vi "INLScan.vi"() -> ()   [LabVIEW 2014]
uses:
  Agilent34401A/FGV.ctl
  Agilent34401A/Agilent34401AData.ctl
  Host API/Controls/FPGA Reference.ctl
  <vilib>/rvi/interface/nirviOpenFPGA/nirviOpenFPGA.xnode
  <vilib>/rvi/interface/nirviMethod/nirviMethod.xnode
  Host API/Controls/SPI Configuration Cluster.ctl
  <vilib>/rvi/interface/nirviCloseFPGA/nirviCloseFPGA.xnode
  FPGA Bitfiles/SPIExample_FPGATarget3_FPGASPIFPGATopLe_SKx8rjJlgp0.lvbitx
  FPGA/FPGA SPI_FPGA Top Level.vi
  <vilib>/rvi/errors/niLvFpgaMergeErrorWithErrorCode.vi
panel:
  out "act rep.":i32
  in  "repetitions":i32
  out "KepcoStep [V]":ext
  out "DAC step [V]":ext format="%#_10g"
  out "StepSize":u32 max=262143 format="%0d"
  out "INL":dbl
  out "Read Data":u8[](array[numeric]) format="%08b"
  out "act Step":u32 format="%018b"
  out "INL":cluster{dbl[], dbl[]}(graph)
  out "last saved":path
  in  "save to":path=path "R:/Projekte/A2-MAINZ-EXP/TRIGA/Measurements and Analysis_Simon/KepcoScans und DAC Scans/DAC - AD5781/20102014/Daten/VOUT_BUF"
  out "Volt measured":cluster{"Measurement":dbl, "VOUT":dbl}(graph)
  out "VOUT":dbl
  in  "VREFN":dbl
  in  "VREFP":dbl
  in  "Stop":bool
  out "error out":errorcluster
  in  "StepSize":u32 max=262143 format="%018b"
  in  "Stop":u32=262143 max=262143 format="%018b"
  out "Volt":dbl
  in  "wait after set (ms)":u32=50
  in  "Adress":refnum<visa-resource-name>="COM1"
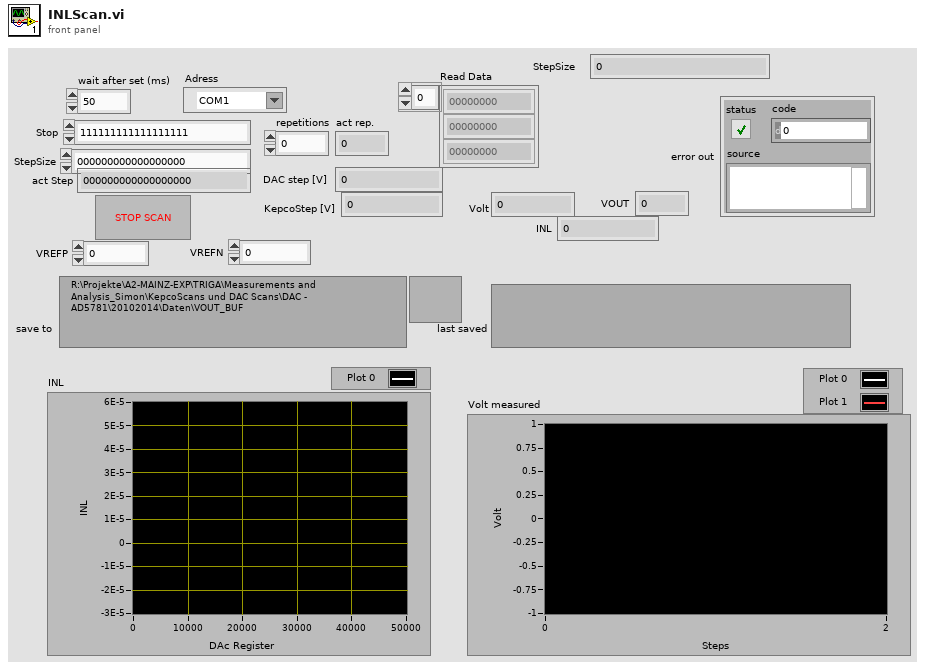
[diagram p1: front panel]
types:
  T1 = typedef "SPI Configuration Cluster.ctl" = cluster{"CS":u8, "Clock Rate (Hz)":dbl, "Clock Mode":u8, "CS Active State":bool}
  T2 = cluster{"Port":i8, "Configuration Cluster":T1, "Hardware Pins":cluster{"RESET":bool, "LDAC":bool, "CLR":bool}, "Total Bits":u16}
  T3 = typedef "Agilent34401AData.ctl" = cluster{"Adress":refnum<visa-resource-name>}
  T4 = typedef "FGV.ctl" = enum16{"Write", "Read", "Init"}
  T5 = typedef "FPGA Reference.ctl" = refnum<k20>
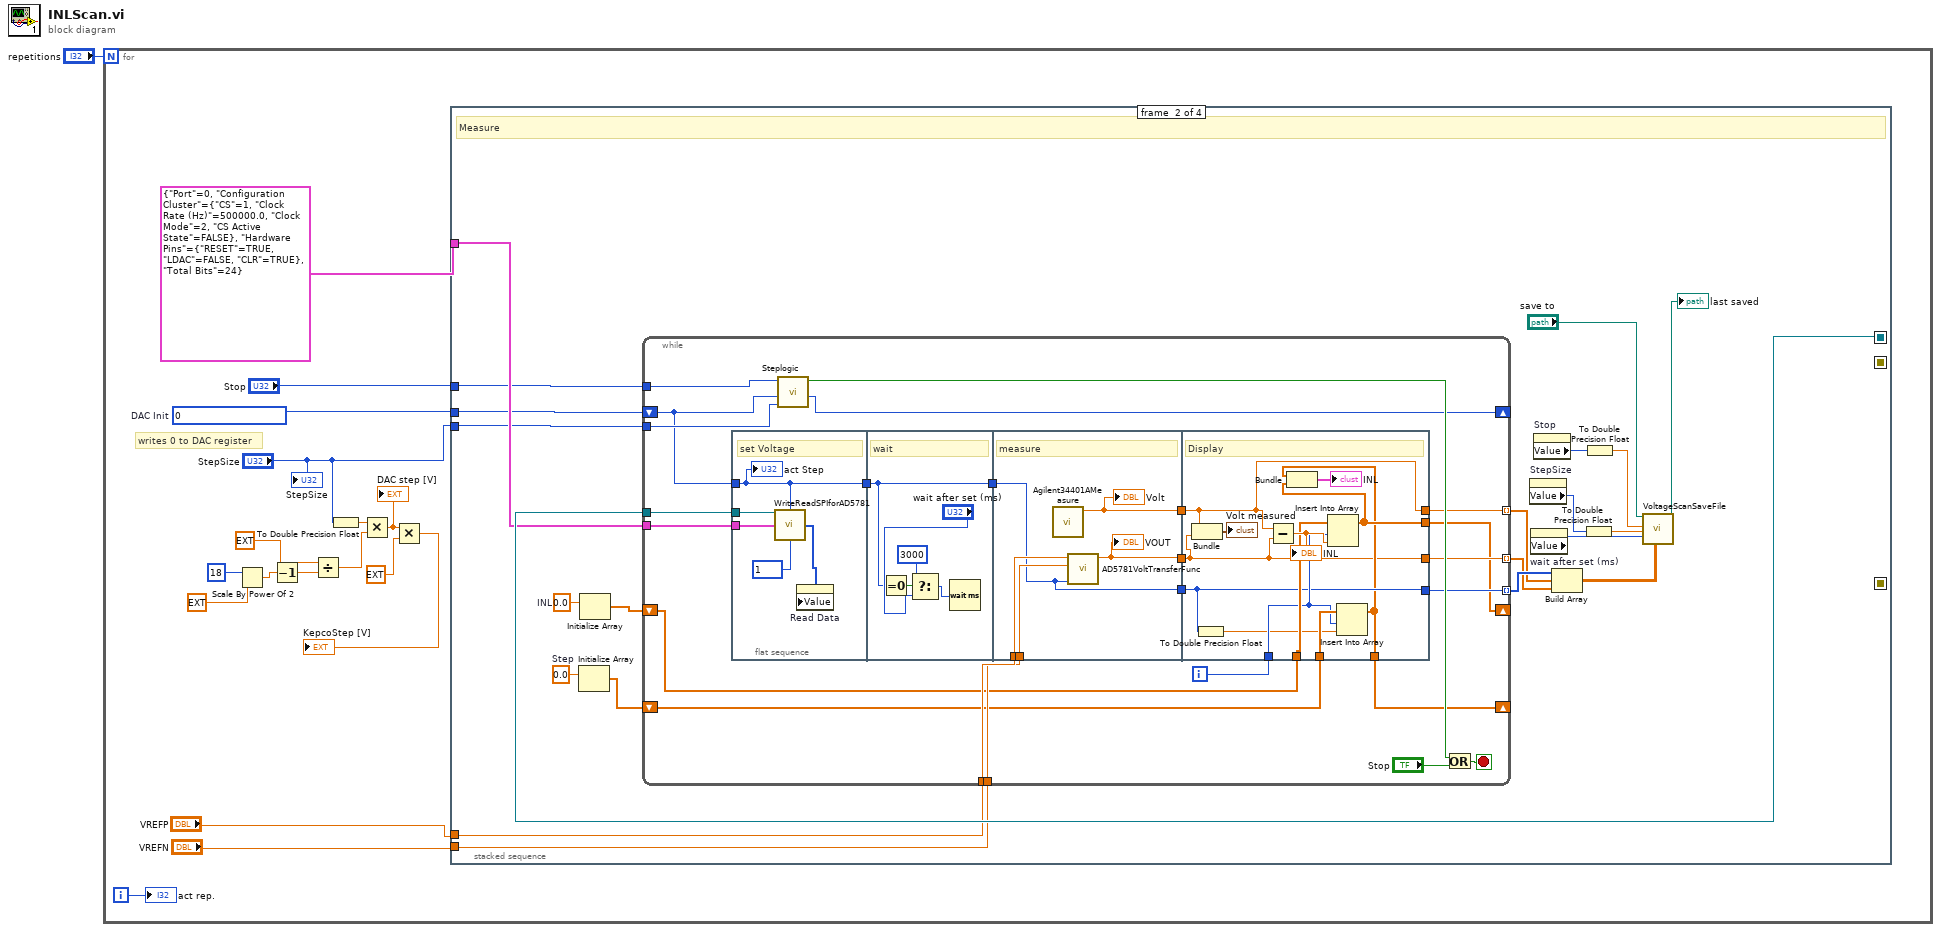
[diagram p0: block diagram]
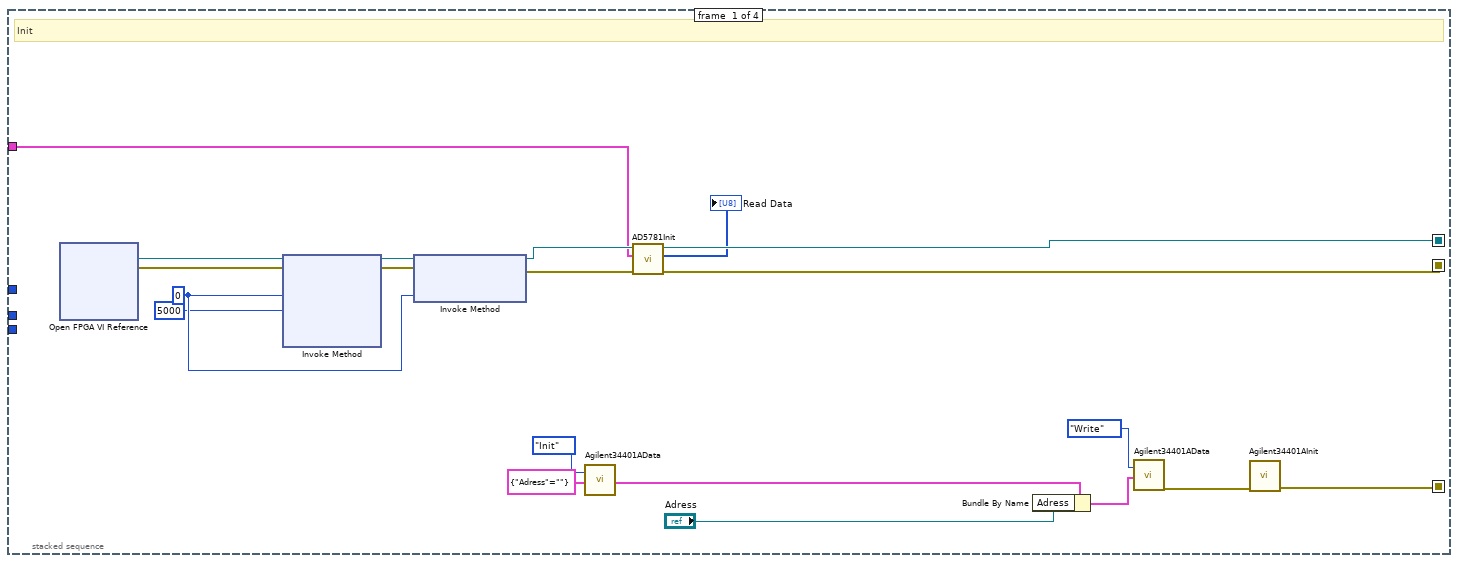
[diagram p2: hidden frame]
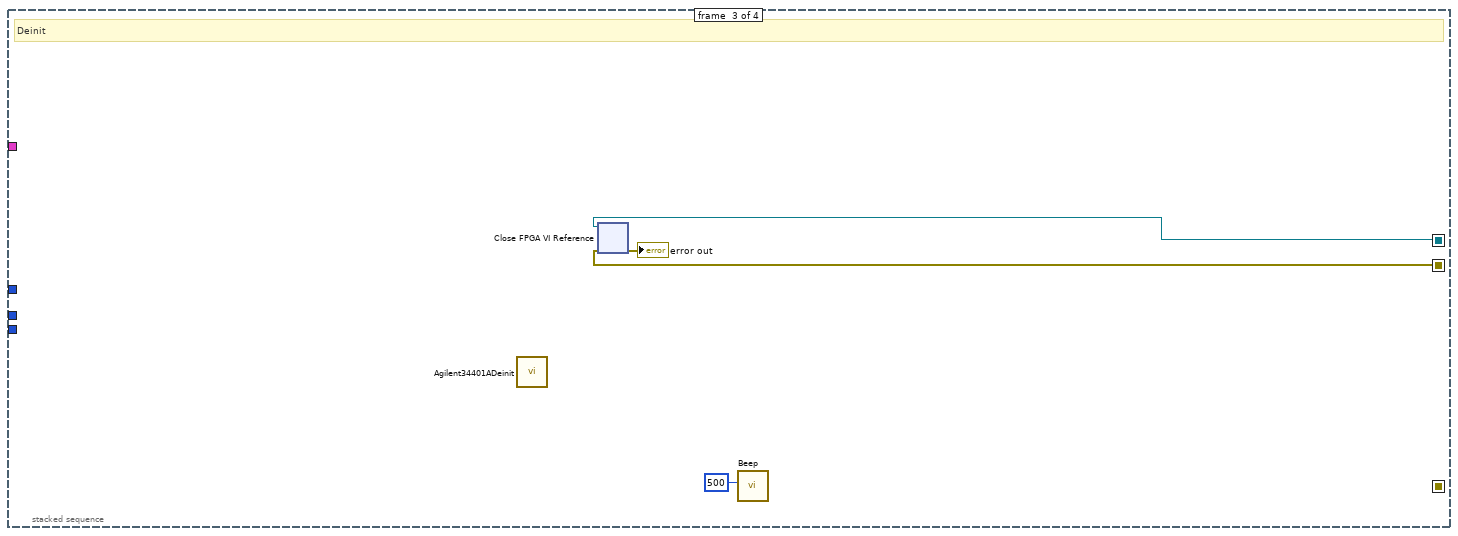
[diagram p3: hidden frame]
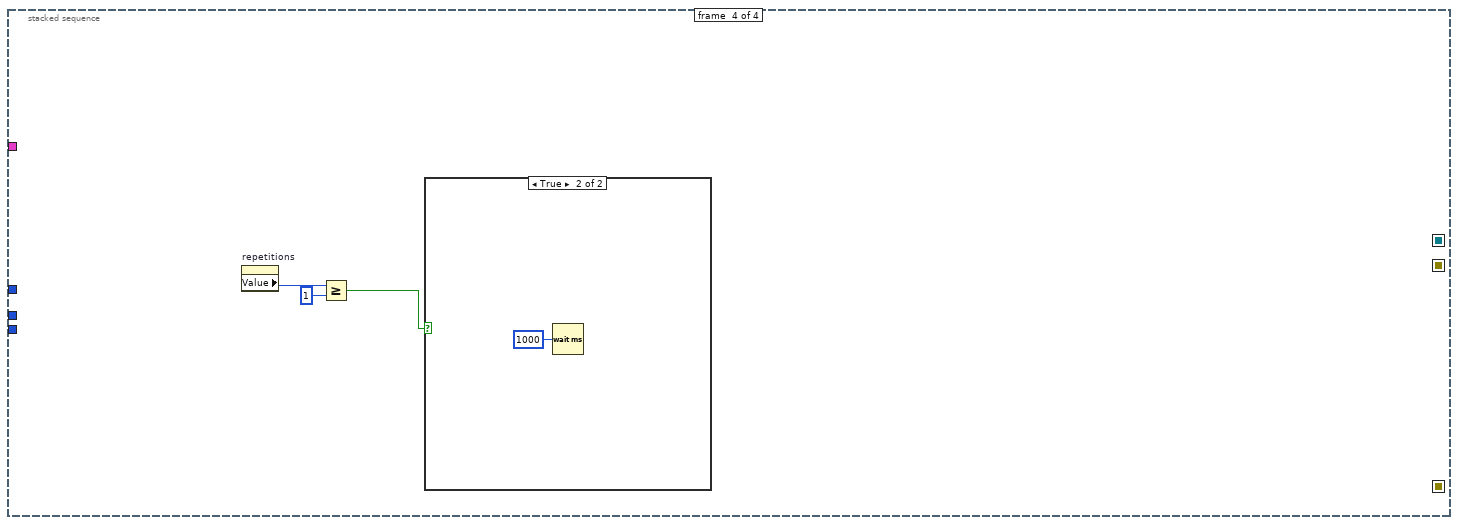
[diagram p4: hidden frame]
diagram:
  n1 = for {
    N: "repetitions" -> [_]
    i -> [w2]
    w17 = u32 0  # DAC Init
    # "writes 0 to DAC register"
    n2 = Scale By Power Of 2(n=i16 18, x=ext 1.0) -> (x*2^n=w9:ext)
    n3 = Decrement(x=w9) -> (x-1=w7:ext)
    n4 = Divide(x=ext 20.0, y=w7) -> (x/y=w6:ext)
    n5 = To Double Precision Float(number="StepSize") -> (double precision float=w12:dbl)
    n6 = Multiply(x=w12, y=w6) -> (x*y=w5:ext)
    "DAC step [V]" <- w5
    n7 = Multiply(x=w5, y=ext 50.0) -> (x*y=→"KepcoStep [V]":ext)
    n8 = stacked-sequence {
      seq-local: [w23 _ _ _] -> [_ w60 w115 _]
      seq-local: [w22 _ _ _] -> [_ _ w114 _]
      seq-local: [w21 _ _ _] -> [_ _ _ _]
      tunnel: T2 {"Port"=0, "Configuration Cluster"={"CS"=1, "Clock Rate (Hz)"=500000.0, "Clock Mode"=2, "CS Active State"=FALSE}, "Hardware Pins"={"RESET"=TRUE, "LDAC"=FALSE, "CLR"=TRUE}, "Total Bits"=24} ("SPI - AD5781 Setup") -> [w20 w59 _ _]
      tunnel: w17 -> [_ w58 _ _]
      tunnel: "Stop" -> [_ w57 _ _]
      tunnel: "StepSize" -> [_ w56 _ _]
      tunnel: "VREFP" -> [_ w55 _ _]
      tunnel: "VREFN" -> [_ w54 _ _]
      frame #0 {
        w31 = 0 ("IRQ Number(s)")
        # "Init"
        n9 = xnode "Open FPGA VI Reference"() -> ("FPGA VI Reference Out"=w26:T5, "error out"=w27:errorcluster)  [unwired: 2 in]
        n10 = xnode "Invoke Method"("FPGA VI Reference In"=w26, "error in"=w27, "IRQ Number(s)"=w31, "Timeout (ms)"=5000) -> ("FPGA VI Reference Out"=w28:T5, "error out"=w29:errorcluster)  [unwired: 2 out]
        n11 = xnode "Invoke Method"("FPGA VI Reference In"=w28, "error in"=w29, "IRQ Number(s)"=w31) -> ("FPGA VI Reference Out"=w24:T5, "error out"=w25:errorcluster)
        n12 = call "Agilent34401AData.vi"("Enum"=FGV."Init", "Cluster"=T3 {"Adress"=""}) -> ("Cluster 2"=w36:T3)  [unwired: 16 in, 1 out]
        n13 = call "AD5781Init.vi"("error in"=w25, "SPI - AD5781 Setup"=w20, "FPGA Interface"=w24) -> ("error out"=w22:errorcluster, "Read Data"=→"Read Data":u8[], "FPGA Interface 2"=w23:T5)  [unwired: 6 in]
        n14 = Bundle By Name(cluster=w36, "Adress"="Adress") -> (w35:T3)
        n15 = call "Agilent34401AData.vi"("Enum"=FGV."Write", "Cluster"=w35) -> ("error out"=w32:errorcluster)  [unwired: 16 in, 1 out]
        n16 = call "Agilent34401AInit.vi"("error in (no error)"=w32) -> ("error out"=w21:errorcluster)  [unwired: 10 in]
      }
      frame #1 {
        w51 = 0.0  # Step
        w53 = 0.0  # INL
        # "Measure"
        n17 = Initialize Array(w51) -> (w50:dbl[])  [unwired: 1 in]
        n18 = Initialize Array(w53) -> (w52:dbl[])  [unwired: 1 in]
        n19 = while {
          tunnel: w60 -> [w84]
          tunnel: w59 -> [w83]
          shift-right: [w81] -> _
          shift-left: w58 -> [w76]
          tunnel: w57 -> [w78]
          tunnel: w56 -> [w77]
          tunnel: w55 -> [w75]
          tunnel: w54 -> [w74]
          tunnel: [w73] -> w49 mode=indexing
          tunnel: [w72] -> w39 mode=indexing
          tunnel: [w71] -> w40 mode=indexing
          shift-right: [w64] -> _
          shift-left: w52 -> [w66]
          shift-right: [w63] -> _
          shift-left: w50 -> [w65]
          i -> [w67]
          stop <- w80 stop-if-true
          n20 = flat-sequence {
            tunnel: w84 -> [w89]
            tunnel: w83 -> [w88]
            tunnel: w76 -> [w85]
            tunnel: [w85] -> w61
            tunnel: [w90] -> w62
            tunnel: w61 -> [w90]
            tunnel: w75 -> [w99]
            tunnel: w74 -> [w98]
            tunnel: [w95] -> w70
            tunnel: [w97] -> w69
            tunnel: [w96] -> w68
            tunnel: w62 -> [w95]
            tunnel: [w102] -> w71
            tunnel: [w101] -> w72
            tunnel: [w107] -> w73
            tunnel: w70 -> [w107]
            tunnel: w69 -> [w101]
            tunnel: w68 -> [w102]
            tunnel: w67 -> [w108]
            tunnel: w66 -> [w110]
            tunnel: w65 -> [w109]
            tunnel: [w104] -> w64
            tunnel: [w103] -> w63
            frame #0 {
              # "set Voltage"
              n21 = call "WriteReadSPIforAD5781.vi"("FPGA VI Reference Out 2"=w89, "DAC 18Bit Data"=w85, "SPI - AD5781 Setup"=w88, "register prefix"=u8 1) -> ("Read Data"=w86:u8[])  [unwired: 9 in, 2 out]
              n22 = property on="Read Data" class="Arr (strict)"("Value"=w86) -> ()  [unwired: 2 in, 2 out]
              "act Step" <- w85
            }
            frame #1 {
              # "wait"
              n23 = Equal To 0?(x=w90) -> (x = 0?=w91:bool)
              n24 = Select(t=u32 3000, s=w91, f="wait after set (ms)") -> (s? t:f=w93:u32)
              n25 = Wait (ms)(milliseconds to wait=w93) -> ()  [unwired: 1 out]
            }
            frame #2 {
              # "measure"
              n26 = call "Agilent34401AMeasure.vi"() -> ("Measurement"=w96:dbl)  [unwired: 10 in, 1 out]
              "Volt" <- w96
              n27 = call "AD5781VoltTransferFunc.vi"("act Step 18 Bit"=w95, "VREFN"=w98, "VREFP"=w99) -> ("VOUT"=w97:dbl)  [unwired: 8 in]
              "VOUT" <- w97
            }
            frame #3 {
              # "Display"
              n28 = Bundle("Measurement"=w102, "VOUT"=w101) -> (→"Volt measured":cluster{"Measurement":dbl, "VOUT":dbl})  [unwired: 1 in]
              n29 = To Double Precision Float(number=w107) -> (double precision float=w106:dbl)
              n30 = Subtract(x=w102, y=w101) -> (x-y=w111:dbl)
              "INL" <- w111
              n31 = Insert Into Array(array=w110, index=w108, new element=w111) -> (w104:dbl[])
              n32 = Insert Into Array(array=w109, index=w108, new element=w106) -> (w103:dbl[])
              n33 = Bundle(w103, w104) -> (→"INL":cluster{dbl[], dbl[]})  [unwired: 1 in]
            }
          }
          n34 = call "Steplogic.vi"("StepSize"=w77, "act Step 18 Bit"=w76, "Stop"=w78) -> ("Next Step"=w81:u32, "Done"=w82:bool)  [unwired: 7 in]
          n35 = Or(x=w82, y="Stop") -> (x .or. y?=w80:bool)
        }
        n36 = property on="StepSize" class="DigNum (strict)"() -> ("Value"=w46:u32)  [unwired: 2 in, 2 out]
        n37 = property on="wait after set (ms)" class="DigNum (strict)"() -> ("Value"=w47:u32)  [unwired: 2 in, 2 out]
        n38 = property on="Stop" class="DigNum (strict)"() -> ("Value"=w44:u32)  [unwired: 2 in, 2 out]
        n39 = Build Array(w49, w40, w39) -> (w48:dbl[][])
        n40 = To Double Precision Float(number=w46) -> (double precision float=w45:dbl)
        n41 = To Double Precision Float(number=w44) -> (double precision float=w43:dbl)
        n42 = call "VoltageScanSaveFile.vi"("Path"="save to", "Stop"=w43, "StepSize/V"=w45, "wait for KepCo"=w47, "array"=w48) -> ("Filename Out"=→"last saved":path)  [unwired: 13 in, 1 out]
      }
      frame #2 {
        # "Deinit"
        n43 = call "Agilent34401ADeinit.vi"() -> ()  [unwired: 11 in, 1 out]
        n44 = xnode "Close FPGA VI Reference"("FPGA VI Reference In"=w115, "error in"=w114) -> ("error out"=→"error out":errorcluster)
        n45 = call <vilib>:"Beep.vi"("duration (msec)"=u32 500) -> ()  [unwired: 11 in]
      }
      frame #3 {
        n46 = property on="repetitions" class="DigNum (strict)"() -> ("Value"=w118:i32)  [unwired: 2 in, 2 out]
        n47 = Greater Or Equal?(x=w118, y=1) -> (x >= y?=w116:bool)
        n48 = case shown="True" w116 {
          frame False {
          }
          frame True {
            n49 = Wait (ms)(milliseconds to wait=u32 1000) -> ()  [unwired: 1 out]
          }
        }
      }
    }
    "StepSize" <- "StepSize"
    "act rep." <- w2
  }
